vi "save standards data.vi"(0 "standard cluster":T1={"Description"="", "Setup"={"integration time"=0.5, "rinse time"=10.0, "sample time"=10.0, "sample type"=0}, "Concentrations"=[], "Absorbance"=[], "Analyst"="", "Concentration units"="", "Good"=[]} {"Absorbance" format="%.2e"; "Concentrations" format="%.3e"; "Setup"."sample type" items=["Sample Cuvet", "Sipper Cell", "No Dialog"]; "Setup"."sample time" min=0.0 max=100.0 step=1.0 format="%.1f"; "Setup"."rinse time" min=0.0 max=100.0 step=1.0 format="%.1f"; "Setup"."integration time" format="%.1f"}) -> ()   [LabVIEW 2015]
uses:
  standard cluster.ctl
  settings.ctl
  file/file action.ctl
panel:
  out "error out":errorcluster
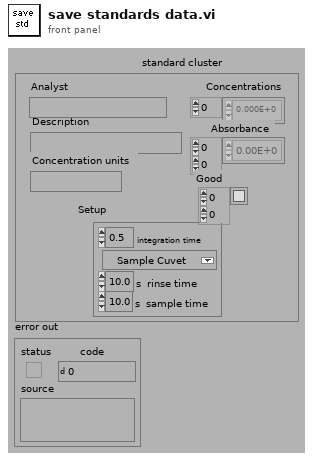
[diagram p1: front panel]
types:
  T1 = typedef "standard cluster.ctl" = cluster{"Description":string, "Setup":T2, "Concentrations":dbl[], "Absorbance":dbl[][], "Analyst":string, "Concentration units":string, "Good":bool[][]}
  T2 = typedef "settings.ctl" = cluster{"integration time":sgl, "rinse time":dbl[unit], "sample time":dbl[unit], "sample type":u16}
  T3 = typedef "file action.ctl" = enum16{"Save", "Open"}
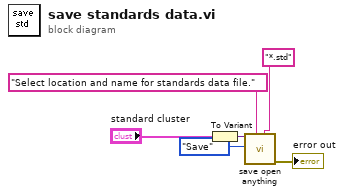
[diagram p0: block diagram]
diagram:
  n1 = To Variant(anything="standard cluster") -> (Variant=w6:variant)
  n2 = call "save open anything.vi"("Variant"=w6, "Action"=file_action."Save", "prompt"="Select location and name for standards data file.", "pattern"="*.std") -> ("error out"=→"error out":errorcluster)  [unwired: 3 in, 3 out]
